vi "1Command-to-JSON.vi"(8 "error in (no error)":errorcluster, 9 "New Type":string, 10 "Name":string, 11 "Command to Send":string) -> (0 "error out":errorcluster, 3 "Command JSON string":string)   [LabVIEW 2017]
uses:
  Common/Typedefs/command.ctl
panel:
  out "Array":string[](array[string])
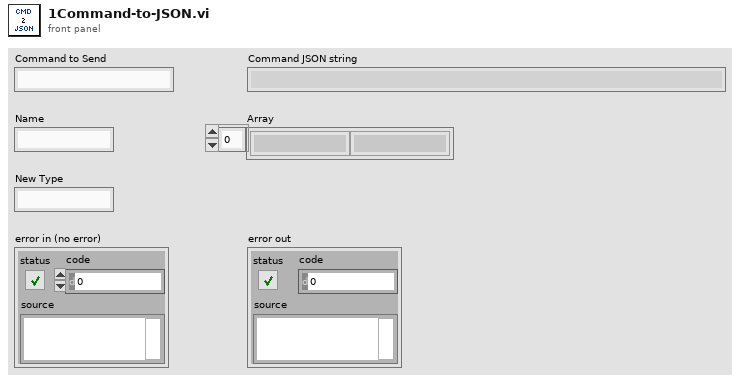
[diagram p1: front panel]
types:
  T1 = typedef "command.ctl" = cluster{"type":string, "command":string, "arguments":string[]}
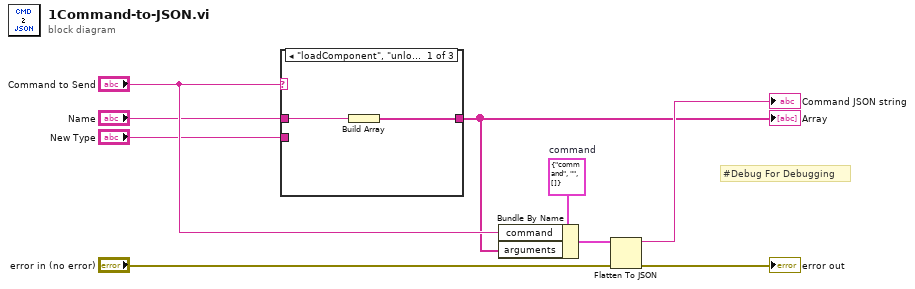
[diagram p0: block diagram]
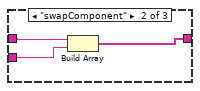
[diagram p2: hidden frame]
diagram:
  w6 = T1 {"type"="command", "command"="", "arguments"=[]}  # command
  # "#Debug For Debugging"
  n1 = case shown="\"loadComponent\", \"unloadComponent\"" "Command to Send" {
    tunnel: "Name" -> [w11 w14 _]
    tunnel: "New Type" -> [_ w12 _]
    tunnel: [w10 w13 _] -> w2
    frame "loadComponent", "unloadComponent" {
      n2 = Build Array(w11) -> (w10:string[])
    }
    frame "swapComponent" {
      n3 = Build Array(w14, w12) -> (w13:string[])
    }
    frame "listActiveComponents", "listComponents", "refresh", Default {
    }
  }
  "Array" <- w2
  n4 = Bundle By Name(cluster=w6, "command"="Command to Send", "arguments"=w2) -> (w5:T1)
  n5 = Flatten To JSON(anything=w5, error in (no error)="error in (no error)") -> (JSON string=→"Command JSON string":string, 11:→"error out":errorcluster)  [unwired: 1 in]
